vi "Destroy.vi"(8 "error in (no error)":errorcluster, 11 "Messenger in":refnum<class "MGR.lvclass">) -> (0 "error out":errorcluster)   [LabVIEW 2011, in "Messenging.lvlib" / "MGR.lvclass"]
uses:
  MGR.lvclass
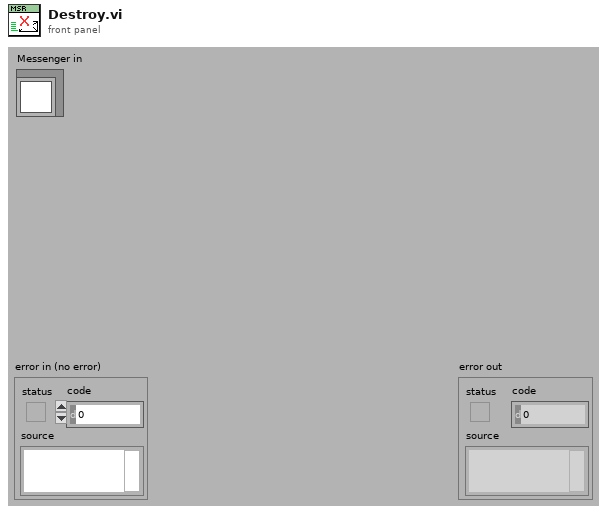
[diagram p1: front panel]
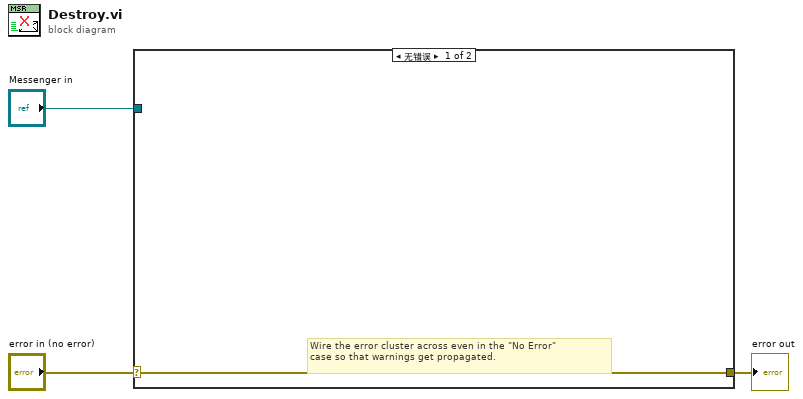
[diagram p0: block diagram]
diagram:
  n1 = case shown="无错误" "error in (no error)" {
    selector: "error in (no error)" -> [w4 w5]
    tunnel: [w4 w5] -> w2
    tunnel: "Messenger in" -> [_ _]
    frame No Error {
      # "Wire the error cluster across even in the \"No Error\"\ncase so that warnings get propagated."
    }
    frame Error {
    }
  }
  "error out" <- w2
